vi "Install Startup.vi"(4 "Version Selection (Exactly)":u32(ring)=1 items=["Highest", "Exactly"], 6 "Uninstall Conflicts (T)":bool=TRUE, 7 "Restart Automatically (T)":bool=TRUE, 8 "error in (no error)":errorcluster, 10 "Startup Application":T1={"title"="", "description"="", "ID"="", "version"="", "component type"=4} {"component type" items=["standard", "hidden", "system", "unknown", "startup", "image"]}, 11 "Session in":refnum<k21>) -> (0 "error out":errorcluster, 1 "Broken Dependencies":T3[](array[typedef]) {"dependee"."component type" items=["standard", "hidden", "system", "unknown", "startup", "image"]; "depender"."component type" items=["standard", "hidden", "system", "unknown", "startup", "image"]}, 2 "Installed Components":T1[](array[typedef]) {"component type" items=["standard", "hidden", "system", "unknown", "startup", "image"]}, 3 "Session out":refnum<k21>, 5 "Uninstalled Components":T1[](array[typedef]) {"component type" items=["standard", "hidden", "system", "unknown", "startup", "image"]})   [LabVIEW 2014, in "nisyscfg.lvlib"]
doc: "Use the Install Startup VI to deploy a startup application to a remote system."
uses:
  nisyscfg.lvlib
  Broken Dependency 1.2.ctl
  Software 1.2.ctl
  Component Type.ctl
  Error Cluster From Error Code.vi
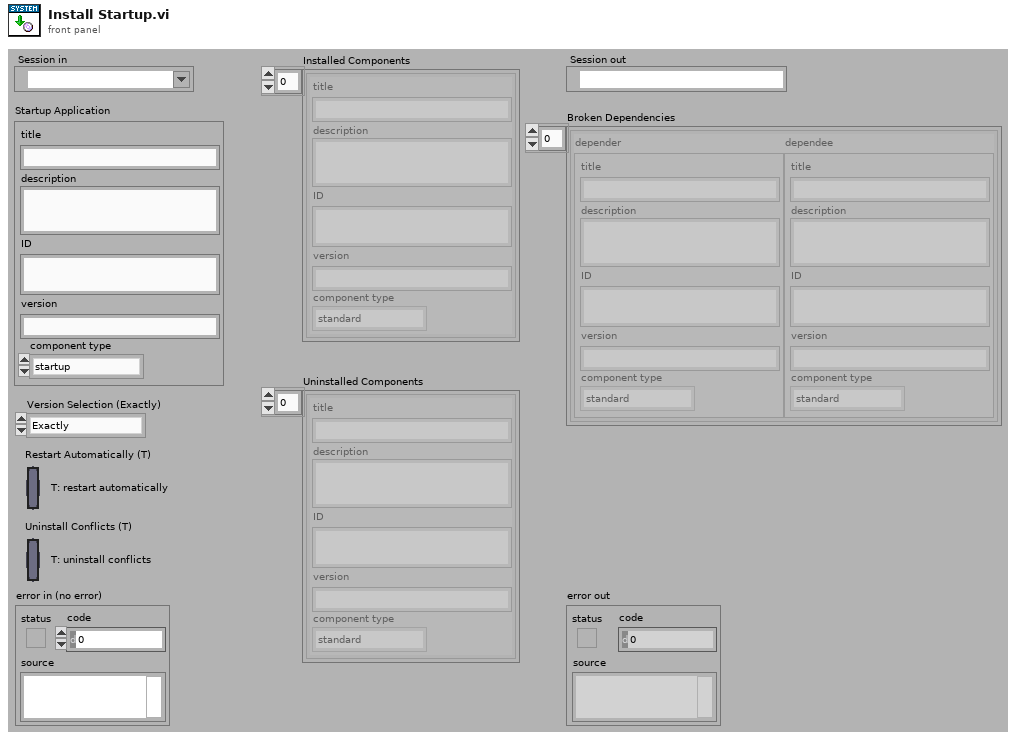
[diagram p1: front panel]
types:
  T1 = typedef "nisyscfg.lvlib/Software 1.2.ctl" = cluster{"title":string, "description":string, "ID":string, "version":string, "component type":T2}
  T2 = typedef "nisyscfg.lvlib/Component Type.ctl" = u32
  T3 = typedef "nisyscfg.lvlib/Broken Dependency 1.2.ctl" = cluster{"depender":T1, "dependee":T1}
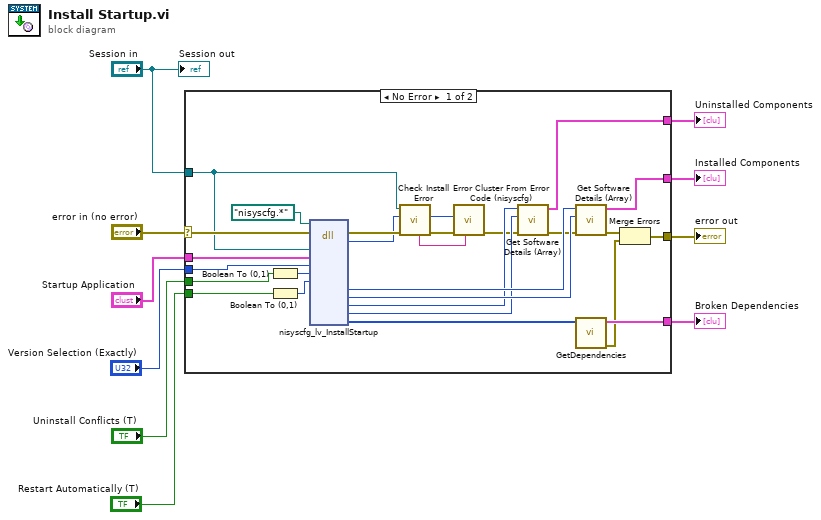
[diagram p0: block diagram]
diagram:
  n1 = case shown="No Error" "error in (no error)" {
    selector: "error in (no error)" -> [w32 w38]
    tunnel: "Session in" -> [w16 _]
    tunnel: [w33 w38] -> w4
    tunnel: [w36 _] -> w5
    tunnel: "Restart Automatically (T)" -> [w31 _]
    tunnel: "Startup Application" -> [w29 _]
    tunnel: "Version Selection (Exactly)" -> [w30 _]
    tunnel: "Uninstall Conflicts (T)" -> [w28 _]
    tunnel: [w24 _] -> w2
    tunnel: [w21 _] -> w1
    frame No Error {
      n2 = Boolean To (0,1)(Boolean=w28) -> (0, 1=w27:i16)
      n3 = Boolean To (0,1)(Boolean=w31) -> (0, 1=w34:i16)
      n4 = dll-call lib="C:/projects/MAX/components/apis/trunk/5.0/objects/scs_nisyscfg_library_dynamic/win32U/i386/msvc90/debug/nisyscfg.dll" fn="nisyscfg_lv_InstallStartup" label="InstallStartup"(path in=path "nisyscfg.*", error in=w32, "session"=w16, "startupComponent"=w29, "versionSelectionMode"=w30, "uninstallConflicts"=w27, "restartAutomatically"=w34) -> (error out=w15:errorcluster, "result"=w14:i32, "installed"=w26:u64, "installedCount"=w25:i32, "uninstalled"=w23:u64, "uninstalledCount"=w22:i32, "brokenDependencies"=w37:u64[])  [unwired: 11 in, 1 out]
      n5 = call "Check Install Error.vi"("error in (no error)"=w15, "Status in"=w14, "Session in"=w16) -> ("error out"=w17:errorcluster, "Status out"=w12:i32, "Details"=w11:string)  [unwired: 5 in, 1 out]
      n6 = call "Error Cluster From Error Code (nisyscfg).vi"("Details String"=w11, "error in (no error)"=w17, "Error Code (0)"=w12) -> ("error out"=w13:errorcluster)  [unwired: 8 in]
      n7 = call "Get Software Details (Array).vi"("error in (no error)"=w13, "Number of Elements"=w22, "Enumerator in"=w23) -> ("error out"=w20:errorcluster, "Software Components"=w21:T1[])  [unwired: 7 in]
      n8 = call "Get Software Details (Array).vi"("error in (no error)"=w20, "Number of Elements"=w25, "Enumerator in"=w26) -> ("error out"=w19:errorcluster, "Software Components"=w24:T1[])  [unwired: 7 in]
      n9 = call "GetDependencies.vi"("Enumerator in"=w37) -> ("error out"=w18:errorcluster, "Dependencies"=w36:T3[])  [unwired: 9 in]
      n10 = Merge Errors(w19, w18) -> (w33:errorcluster)
    }
    frame Error {
    }
  }
  "error out" <- w4
  "Broken Dependencies" <- w5
  "Installed Components" <- w2
  "Uninstalled Components" <- w1
  "Session out" <- "Session in"
